vi "_Parse DBL Array Result.vi"(8 "error in (no error)":errorcluster, 10 "Input String":string, 11 "VISA resource name":refnum<visa-resource-name>) -> (0 "error out":errorcluster, 1 "Results":dbl[](array[numeric]) format="%^.3e", 2 "Reliability":i32, 3 "VISA resource name out":refnum<visa-resource-name>)   [LabVIEW 2020, in "Rohde&Schwarz CMWXP NR FR1 Measurement.lvlib"]
uses:
  <instrlib>/Rohde&Schwarz CMWXP NR FR1 Measurement/Rohde&Schwarz CMWXP NR FR1 Measurement.lvlib
  <instrlib>/Rohde&Schwarz CMWXP NR FR1 Measurement/Private/rsidr_core.llb/rsidr_core.lvlib
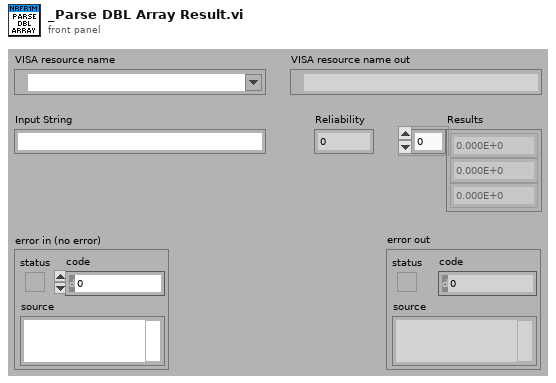
[diagram p1: front panel]
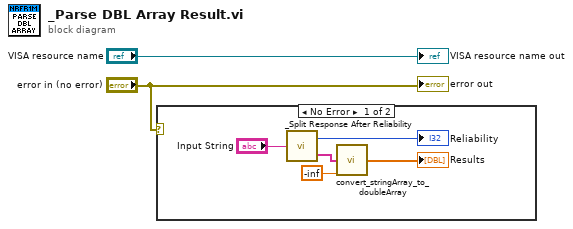
[diagram p0: block diagram]
diagram:
  n1 = case shown="No Error" "error in (no error)" {
    frame No Error {
      n2 = call <instrlib>:"_Split Response After Reliability.vi"("Input String"="Input String") -> ("Response out"=w5:string[], "Reliability out"=→"Reliability":i32)
      n3 = call <instrlib>:"convert_stringArray_to_doubleArray.vi"("default (0)"=-inf, "string array in"=w5) -> ("double array out"=→"Results":dbl[])  [unwired: 3 in]
    }
    frame Error {
    }
  }
  "VISA resource name out" <- "VISA resource name"
  "error out" <- "error in (no error)"
